vi "measure down hole pressure and save to csv file.vi"(0 "Path in":refnum<vi>, 1 "reference 3":refnum<vi>, 2 "reference in":refnum<vi>, 5 "reference 4":refnum<vi>, 7 "reference 5":refnum<vi>, 9 "Record DTW File":bool, 11 "error in (no error)":errorcluster, 12 "Array in":refnum<k24>[](array[refnum]), 13 "Input Variables and Slopes":T1 {"Aux 3 Slope" format="%.2f"; "Aux 2 Slope" format="%.2f"; "Aux 1 Slope" format="%.2f"; "Up Hole  Pressure Offset" format="%.2f"; "DH Pressure Offset" format="%.2f"; "DH Pressure Trans Slope" format="%.2f"; "Height of Sample Box" format="%.2f"; "Reservoir Pressure" format="%.2f"; "Atmospheric Pressure" format="%.2f"; "Depth to Water Table" format="%.2f"; "Up Hole Pressure Slope" format="%.2f"; "Flow Slope" format="%.2f"; "String Pot Slope" format="%.2f"; "Total Volume" format="%.2f"}) -> (4 "DTW path 2":path, 6 "Array out":refnum<k24>[](array[refnum]), 8 "In-Line Pressure":dbl format="%.2f", 15 "error out":errorcluster)   [LabVIEW 2016]
uses:
  Control 2.ctl
  C:/Program Files (x86)/National Instruments/LabVIEW 2016/vi.lib/ULx/ULx_LV.dll
  Kpro Globals.vi
  <userlib>/_OpenG.lib/file/file.llb/Strip Path - Traditional__ogtk.vi
  <userlib>/_OpenG.lib/file/file.llb/Build Path - Traditional__ogtk.vi
  <vilib>/Utility/file.llb/Write Delimited Spreadsheet (DBL).vi
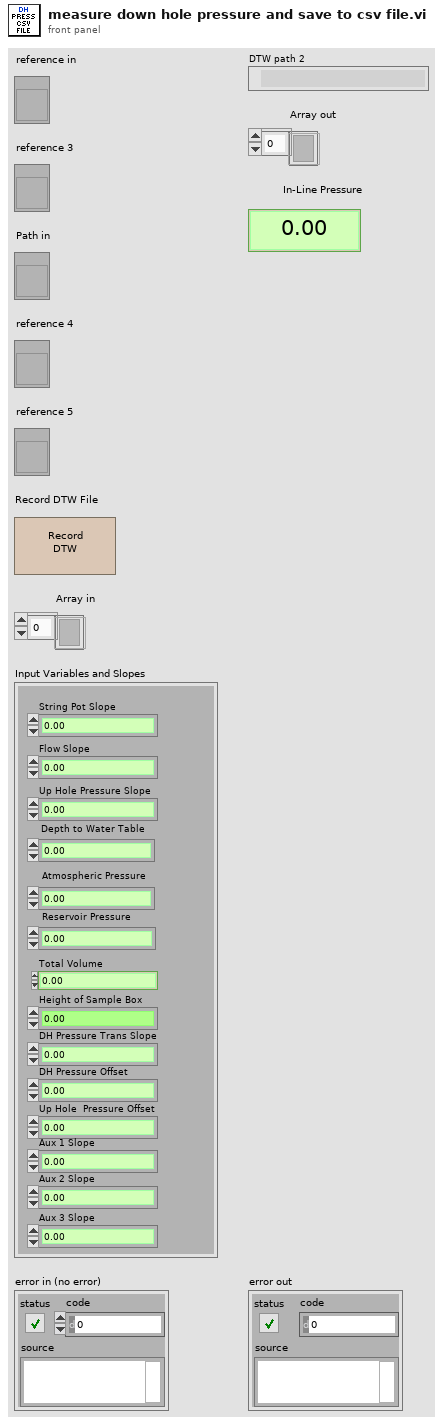
[diagram p1: front panel]
types:
  T1 = typedef "Control 2.ctl" = cluster{"Total Volume":dbl, "String Pot Slope":dbl, "Flow Slope":dbl, "Up Hole Pressure Slope":dbl, "Depth to Water Table":dbl, "Atmospheric Pressure":dbl, "Reservoir Pressure":dbl, "Height of Sample Box":dbl, "DH Pressure Trans Slope":dbl, "DH Pressure Offset":dbl, "Up Hole  Pressure Offset":dbl, "Aux 1 Slope":dbl, "Aux 2 Slope":dbl, "Aux 3 Slope":dbl}
  T2 = typedef "MCC DAQ Readings.ctl" = cluster{"Uphole Pressure":dbl, "Flow":dbl, "Downhole Pressure":dbl, "Top String Pot":dbl, "String Pot":dbl, "Aux 1":dbl, "Aux 2":dbl, "Aux 3":dbl, "9V Monitor":dbl}
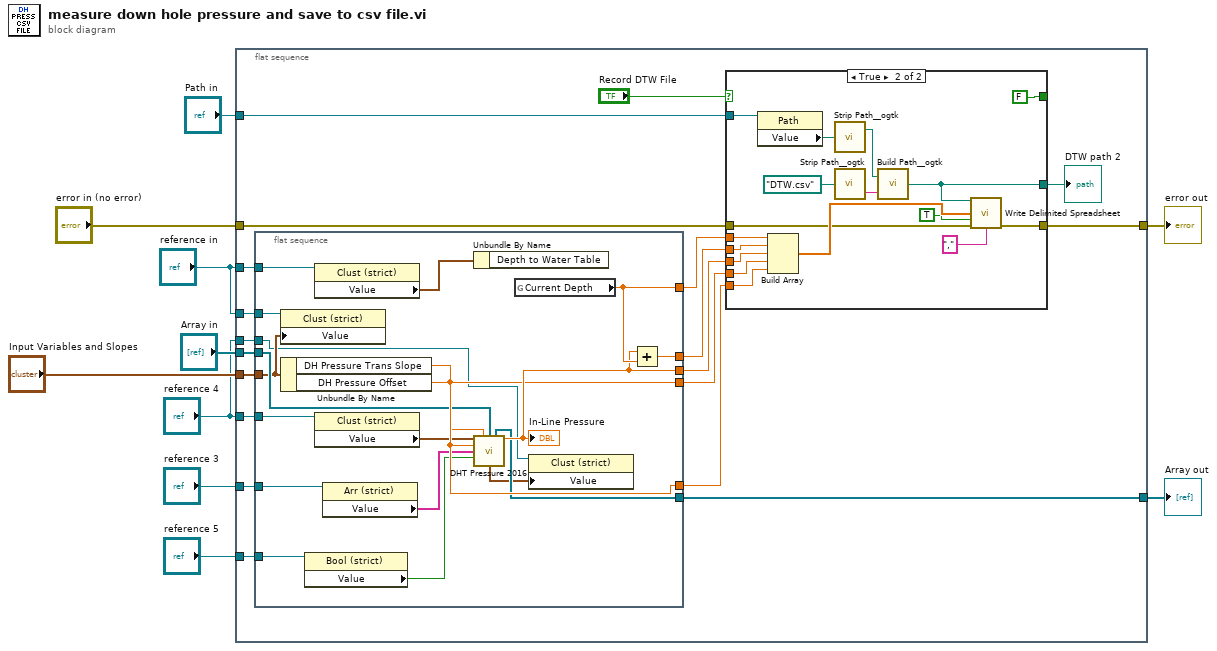
[diagram p0: block diagram]
diagram:
  n1 = flat-sequence {
    tunnel: "Array in" -> [w23]
    tunnel: [w22] -> w7
    tunnel: "Input Variables and Slopes" -> [w21]
    tunnel: "error in (no error)" -> [w20]
    tunnel: [w19] -> w10
    tunnel: "Path in" -> [w17]
    tunnel: "reference in" -> [w16]
    tunnel: "reference 3" -> [w15]
    tunnel: "reference 4" -> [w14]
    tunnel: "reference 4" -> [w13]
    tunnel: "reference 5" -> [w12]
    tunnel: "reference in" -> [w11]
    frame #0 {
      n2 = flat-sequence {
        tunnel: [w48] -> w29
        tunnel: [w47] -> w27
        tunnel: [w46] -> w26
        tunnel: [w45] -> w25
        tunnel: [w44] -> w24
        tunnel: w23 -> [w43]
        tunnel: [w42] -> w22
        tunnel: w21 -> [w38]
        tunnel: w16 -> [w35]
        tunnel: w15 -> [w34]
        tunnel: w14 -> [w33]
        tunnel: w13 -> [w32]
        tunnel: w12 -> [w31]
        tunnel: w11 -> [w30]
        frame #0 {
          n3 = property class="Clust (strict)"(reference=w35, "Value"=w38) -> ()  [unwired: 1 in, 2 out]
          n4 = Unbundle By Name(w38) -> ("DH Pressure Trans Slope"=w45:dbl, "DH Pressure Offset"=w44:dbl)
          n5 = property class="Bool (strict)"(reference=w31) -> ("Value"=w37:bool)  [unwired: 1 in, 2 out]
          n6 = property class="Clust (strict)"(reference=w30) -> ("Value"=w36:T1)  [unwired: 1 in, 2 out]
          n7 = property class="Clust (strict)"(reference=w33) -> ("Value"=w40:T2)  [unwired: 1 in, 2 out]
          n8 = property class="Arr (strict)"(reference=w34) -> ("Value"=w41:string[])  [unwired: 1 in, 2 out]
          n9 = Unbundle By Name(w36) -> ()  [unwired: 1 out]
          n10 = call "DHT Pressure 2016.vi"("Sensor Cluster"=w40, "DHT Pressure Offset"=w44, "Array in"=w43, "DHT Pressure \nSlope"=w45, "Descriptions"=w41, "Zero Pressure\n(F = leave as is)"=w37) -> ("Array out"=w42:refnum<k24>[], "DHT Pressure"=w46:dbl, "Sensor Cluster 2"=w39:T2)  [unwired: 7 in]
          "In-Line Pressure" <- w46
          n11 = global read "Kpro Globals.vi" "Current Depth"() -> (w48:sgl)
          n12 = property class="Clust (strict)"(reference=w32, "Value"=w39) -> ()  [unwired: 1 in, 2 out]
          n13 = Add(x=w46, y=w48) -> (x+y=w47:dbl)
        }
      }
      n14 = case shown="True" "Record DTW File" {
        selector: "Record DTW File" -> [w50 _]
        tunnel: [w50 FALSE ("Boolean")] -> _
        tunnel: w27 -> [_ w63]
        tunnel: w29 -> [_ w64]
        tunnel: w24 -> [_ w61]
        tunnel: w26 -> [_ w62]
        tunnel: w25 -> [_ w60]
        tunnel: w20 -> [w49 w55]
        tunnel: [w49 w54] -> w19
        tunnel: [_ w52] -> w18
        tunnel: w17 -> [_ w51]
        frame False {
        }
        frame True {
          n15 = property class="Path"(reference=w51) -> ("Value"=w59:path)  [unwired: 1 in, 2 out]
          n16 = Build Array(w64, w63, w62, w61, w60) -> (w67:dbl[])
          n17 = call-poly <userlib>:"Strip Path__ogtk.vi"("path"=w59) -> ("stripped path"=w58:path)  [unwired: 1 out]
          n18 = call-poly <userlib>:"Strip Path__ogtk.vi"("path"=path "DTW.csv") -> ("name"=w56:string)  [unwired: 1 out]
          n19 = call-poly <userlib>:"Build Path__ogtk.vi"("name or relative path"=w56, "base path"=w58) -> ("appended path"=w52:path)
          n20 = call-poly <vilib>:"Write Delimited Spreadsheet.vi"("file path (dialog if empty)"=w52, "1D data"=w67, "append to file? (new file:F)"=TRUE, "error in (no error)"=w55, "delimiter (\\t)"="," ("delimiter (\\t)")) -> ("error out"=w54:errorcluster)  [unwired: 9 in, 1 out]
        }
      }
      "DTW path 2" <- w18
    }
  }
  "error out" <- w10
  "Array out" <- w7
